vi "Variant to [I64].vi"(2 "Variant":variant) -> (7 "Value":i64[](array[numeric]))   [LabVIEW 2019, in "Variant to Data.lvlib"]
uses:
  Variant to Data.lvlib
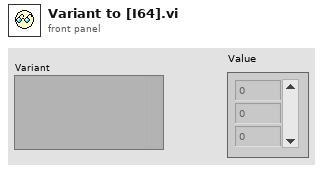
[diagram p1: front panel]
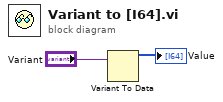
[diagram p0: block diagram]
diagram:
  n1 = Variant To Data(Variant="Variant") -> (data=→"Value":i64[])  [unwired: 2 in, 1 out]
